vi "Update controls.vi"(8 "error in (no error)":errorcluster caption="entrée d'erreur (pas d'erreur)", 10 "IHM Data refnum":T1, 11 "Front Panel status":T2) -> (0 "error out":errorcluster caption="sortie d'erreur")   [LabVIEW 2017, in "IHM Control.lvlib"]
doc: "Le VI Update Controls, permet la modification de l'affichage des bouton de la face avant du programme Main."
uses:
  IHM Control.lvlib
  Front Panel Status.ctl
  MHL UI Ref.ctl
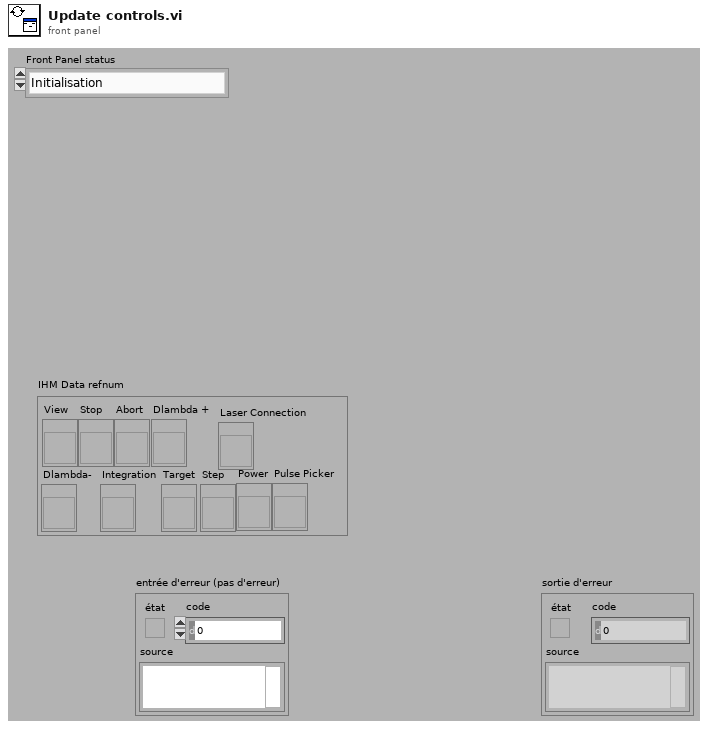
[diagram p1: front panel]
types:
  T1 = typedef "IHM Control.lvlib/MHL UI Ref.ctl" = cluster{"Dlambda-":refnum<vi>, "Abort":refnum<vi>, "Dlambda +":refnum<vi>, "Stop":refnum<vi>, "View":refnum<vi>, "Integration":refnum<vi>, "Target ":refnum<vi>, "Step ":refnum<vi>, "Laser Connection":refnum<vi>, "Power":refnum<vi>, "Pulse Picker":refnum<vi>}
  T2 = typedef "IHM Control.lvlib/Front Panel Status.ctl" = enum16{"Initialisation", "Enable Slit", "Enable Positionner", "Enable Spectrometer", "Enable Laser", "Disable Slit", "Disable Positionner", "Disable Spectrometer", "Disable Laser"}
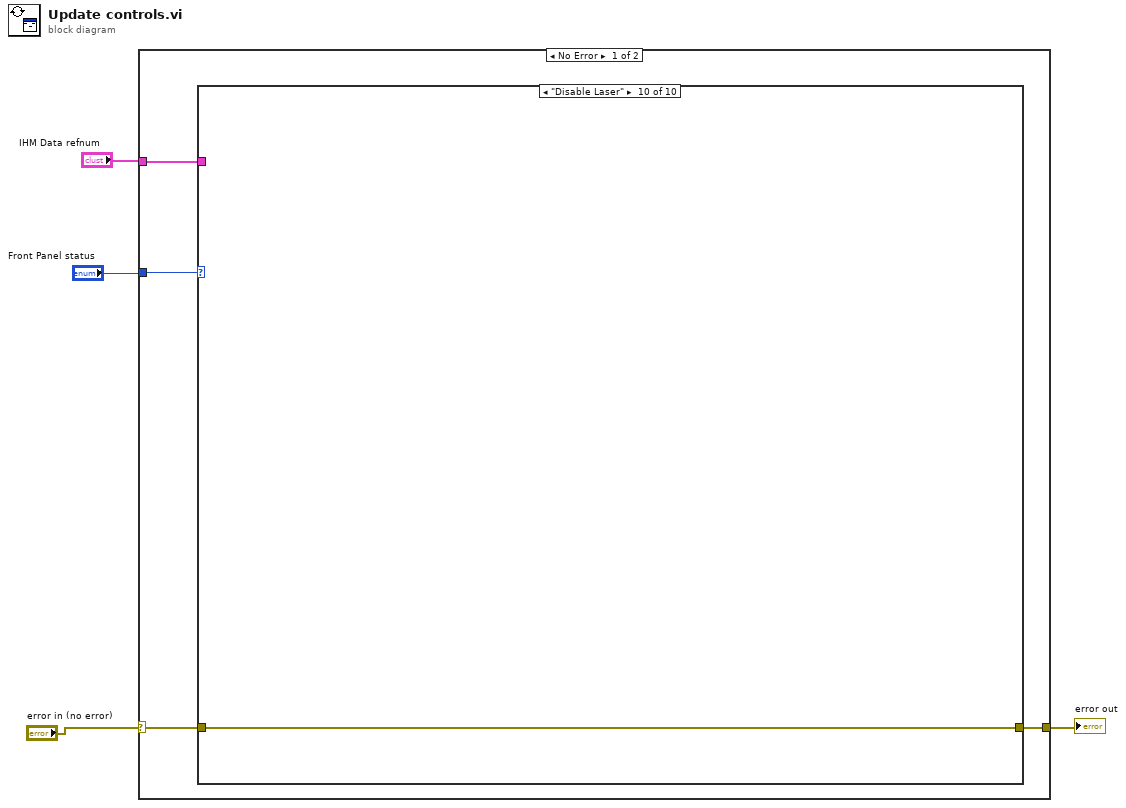
[diagram p0: block diagram]
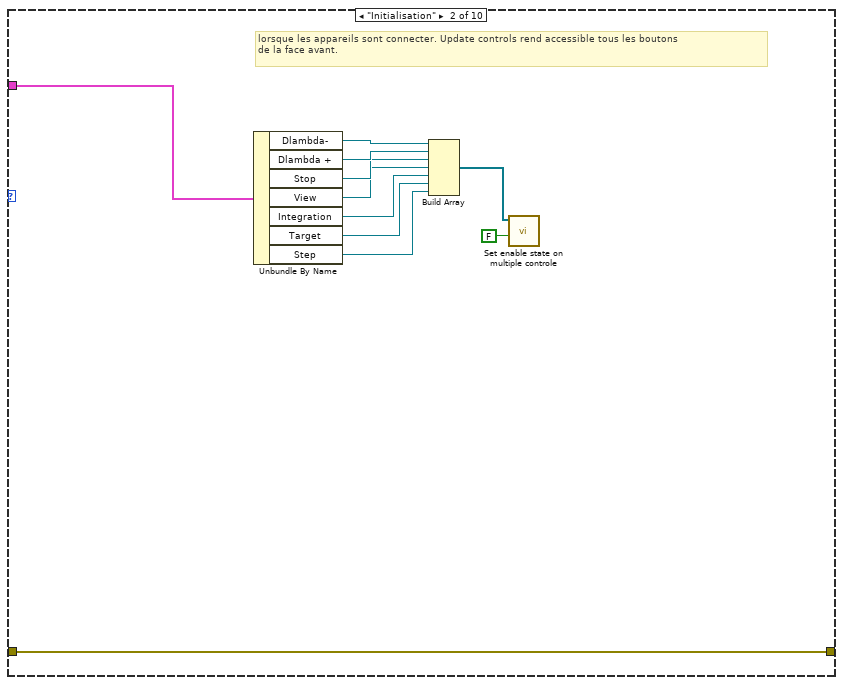
[diagram p3: hidden frame]
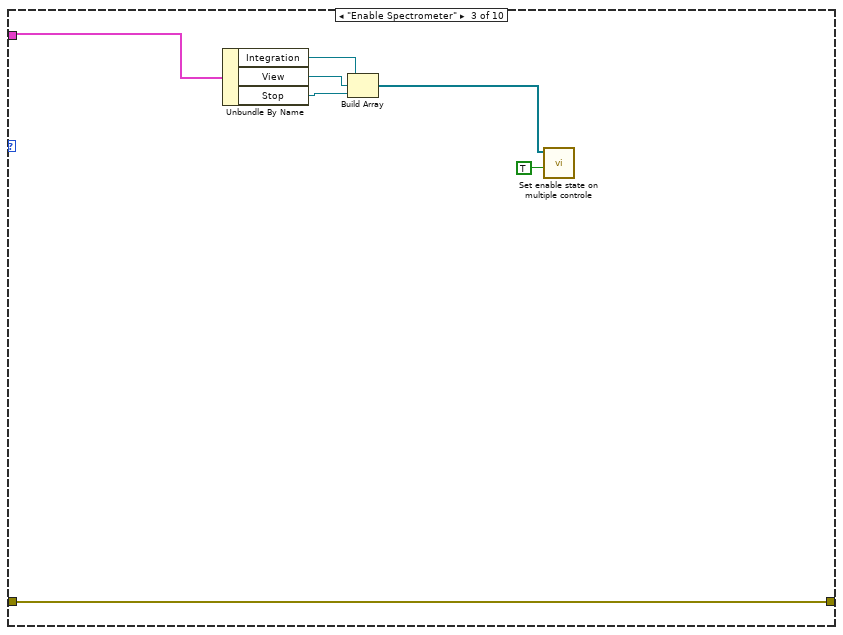
[diagram p4: hidden frame]
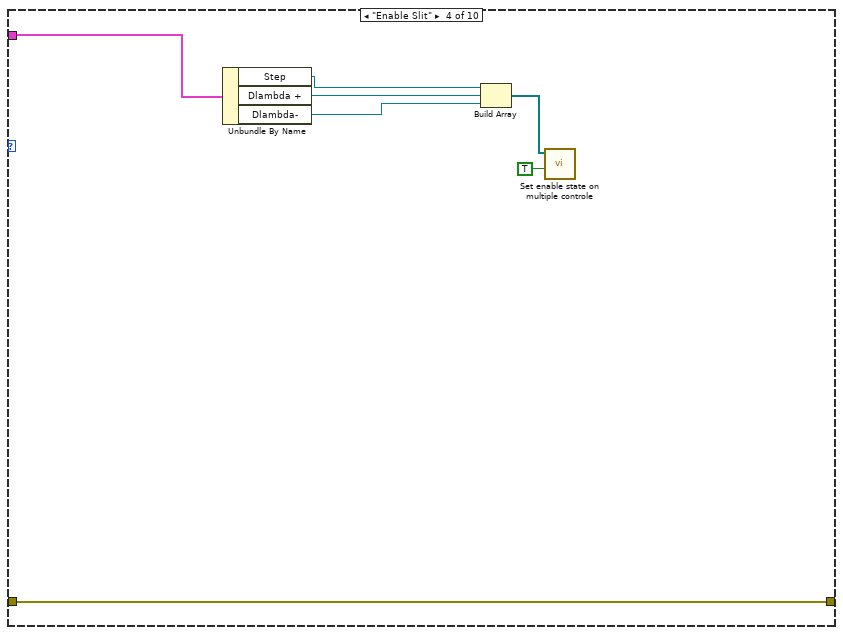
[diagram p5: hidden frame]
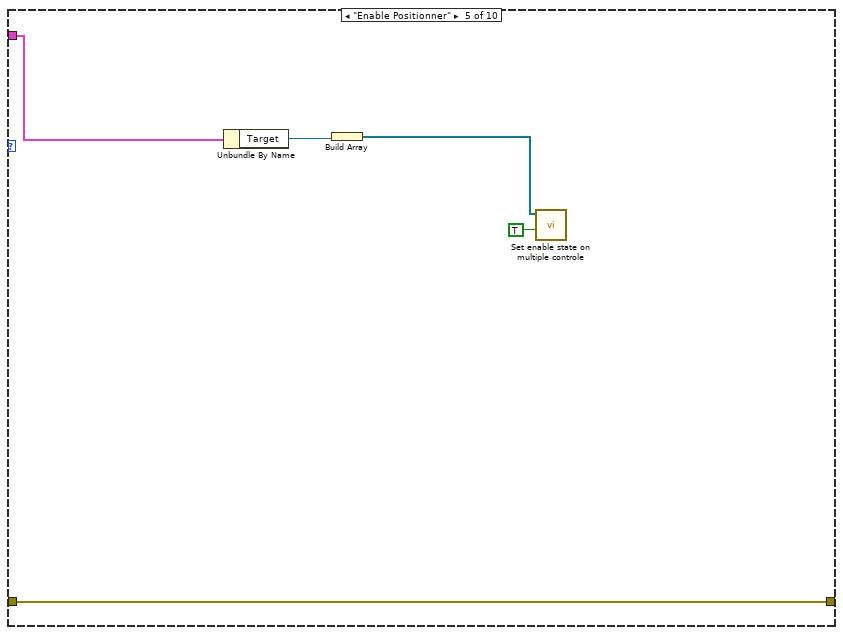
[diagram p6: hidden frame]
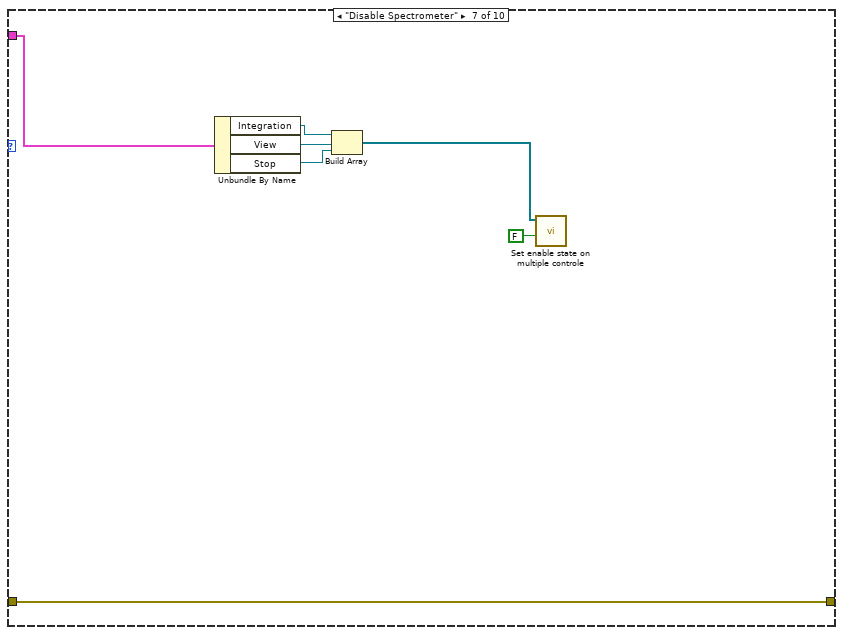
[diagram p8: hidden frame]
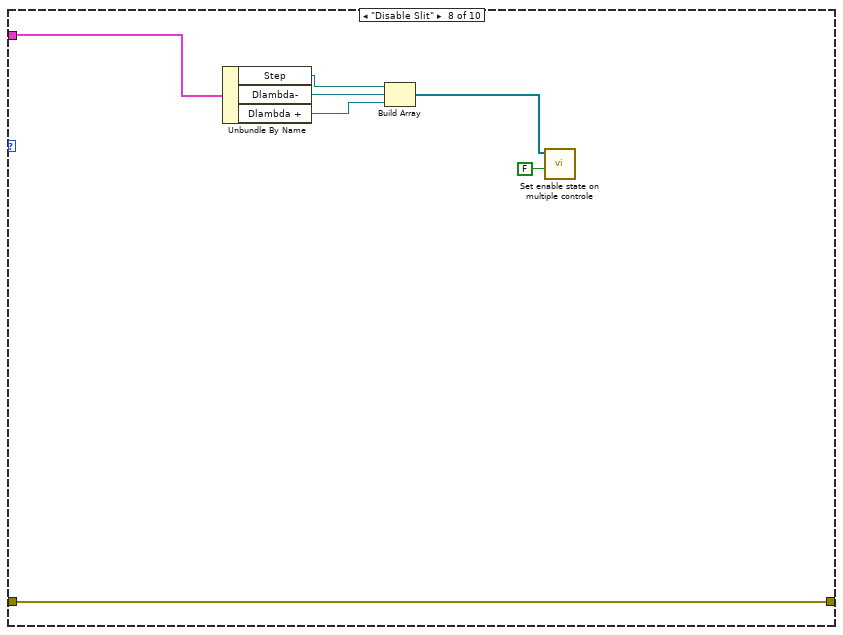
[diagram p9: hidden frame]
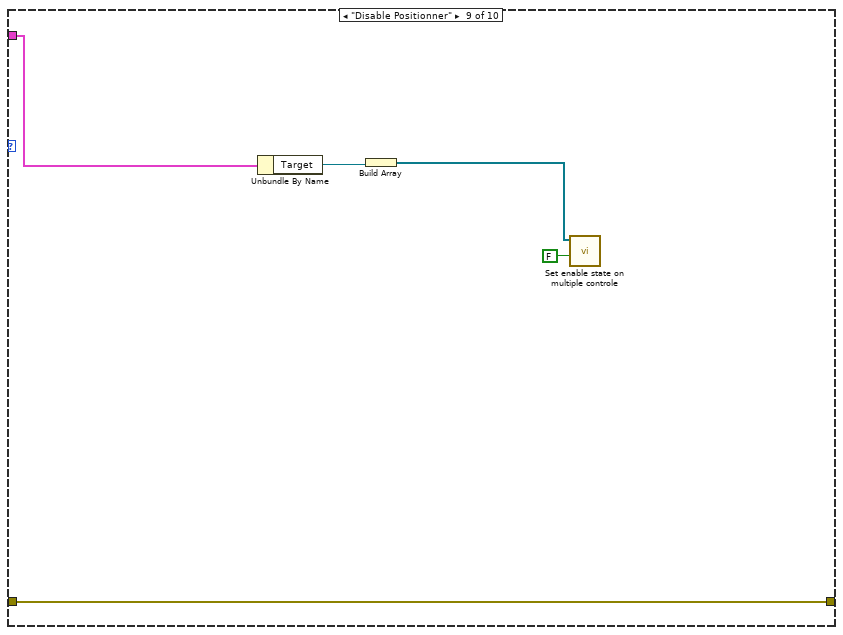
[diagram p10: hidden frame]
diagram:
  n1 = case shown="No Error" "error in (no error)" {
    selector: "error in (no error)" -> [w6 w61]
    tunnel: "Front Panel status" -> [w8 _]
    tunnel: "IHM Data refnum" -> [w7 _]
    tunnel: [w5 w61] -> w2
    frame No Error {
      n2 = case shown="\"Disable Laser\"" w8 {
        tunnel: w7 -> [_ w20 w25 w29 w35 _ w42 w52 w55 _]
        tunnel: [w9 w19 w27 w34 w39 w40 w47 w54 w59 w60] -> w5
        tunnel: w6 -> [w9 w19 w27 w34 w39 w40 w47 w54 w59 w60]
        frame Default {
        }
        frame "Initialisation" {
          # "lorsque les appareils sont connecter. Update controls rend accessible tous les boutons\nde la face avant."
          n3 = Unbundle By Name(w20) -> ("Dlambda-"=w17:refnum<vi>, "Dlambda +"=w16:refnum<vi>, "Stop"=w15:refnum<vi>, "View"=w14:refnum<vi>, "Integration"=w13:refnum<vi>, "Target"=w12:refnum<vi>, "Step"=w11:refnum<vi>)
          n4 = Build Array(w17, w16, w15, w14, w13, w12, w11) -> (w10:refnum<vi>[])
          n5 = call "Set enable state on multiple controle.vi"("Booléen"=FALSE, "Ref. Tab"=w10) -> ()  [unwired: 10 in]
        }
        frame "Enable Spectrometer" {
          n6 = Unbundle By Name(w25) -> ("Integration"=w21:refnum<vi>, "View"=w22:refnum<vi>, "Stop"=w24:refnum<vi>)
          n7 = Build Array(w21, w22, w24) -> (w23:refnum<vi>[])
          n8 = call "Set enable state on multiple controle.vi"("Booléen"=TRUE, "Ref. Tab"=w23) -> ()  [unwired: 10 in]
        }
        frame "Enable Slit" {
          n9 = Unbundle By Name(w29) -> ("Step"=w28:refnum<vi>, "Dlambda +"=w32:refnum<vi>, "Dlambda-"=w31:refnum<vi>)
          n10 = Build Array(w28, w32, w31) -> (w30:refnum<vi>[])
          n11 = call "Set enable state on multiple controle.vi"("Booléen"=TRUE, "Ref. Tab"=w30) -> ()  [unwired: 10 in]
        }
        frame "Enable Positionner" {
          n12 = Unbundle By Name(w35) -> ("Target"=w37:refnum<vi>)
          n13 = Build Array(w37) -> (w38:refnum<vi>[])
          n14 = call "Set enable state on multiple controle.vi"("Booléen"=TRUE, "Ref. Tab"=w38) -> ()  [unwired: 10 in]
        }
        frame "Enable Laser" {
        }
        frame "Disable Spectrometer" {
          n15 = Unbundle By Name(w42) -> ("Integration"=w41:refnum<vi>, "View"=w45:refnum<vi>, "Stop"=w44:refnum<vi>)
          n16 = Build Array(w41, w45, w44) -> (w43:refnum<vi>[])
          n17 = call "Set enable state on multiple controle.vi"("Booléen"=FALSE, "Ref. Tab"=w43) -> ()  [unwired: 10 in]
        }
        frame "Disable Slit" {
          n18 = Unbundle By Name(w52) -> ("Step"=w51:refnum<vi>, "Dlambda-"=w50:refnum<vi>, "Dlambda +"=w49:refnum<vi>)
          n19 = Build Array(w51, w50, w49) -> (w48:refnum<vi>[])
          n20 = call "Set enable state on multiple controle.vi"("Booléen"=FALSE, "Ref. Tab"=w48) -> ()  [unwired: 10 in]
        }
        frame "Disable Positionner" {
          n21 = Unbundle By Name(w55) -> ("Target"=w57:refnum<vi>)
          n22 = Build Array(w57) -> (w58:refnum<vi>[])
          n23 = call "Set enable state on multiple controle.vi"("Booléen"=FALSE, "Ref. Tab"=w58) -> ()  [unwired: 10 in]
        }
        frame "Disable Laser" {
        }
      }
    }
    frame Error {
    }
  }
  "error out" <- w2
